vi "Aim X&Y Compre.vi"(10 "Y":i64, 11 "X":i64) -> (3 "X&Y cordinate":dbl)   [LabVIEW 2020]
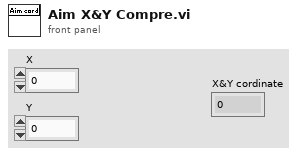
[diagram p1: front panel]
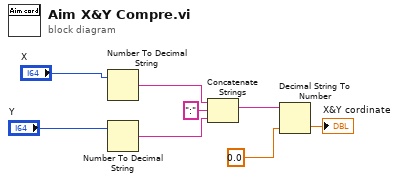
[diagram p0: block diagram]
diagram:
  n1 = Number To Decimal String(number="X") -> (decimal integer string=w6:string)  [unwired: 1 in]
  n2 = Number To Decimal String(number="Y") -> (decimal integer string=w4:string)  [unwired: 1 in]
  n3 = Concatenate Strings(w6, ":" ("string"), w4) -> (w3:string)
  n4 = Decimal String To Number(string=w3, default (0L)=0.0) -> (number=→"X&Y cordinate":dbl)  [unwired: 1 in, 1 out]
